vi "Delete Source Files Missing From Install.vi"(8 "Error In":errorcluster, 10 "Source Files":path[](array[path]), 11 "Configuration":T1) -> (0 "Error Out":errorcluster, 2 "Deleted From Souce":path[](array[path]), 3 "Configuration":T1)   [LabVIEW 2011, in "LVH-Build-Tools.lvlib"]
uses:
  LVH-Build-Tools.lvlib
  Type Defs/Configuration.ctl
  Type Defs/Install Configuration.ctl
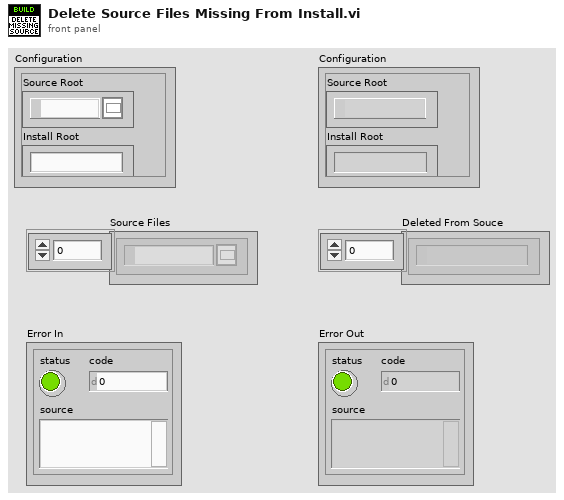
[diagram p1: front panel]
types:
  T1 = typedef "LVH-Build-Tools.lvlib/Configuration.ctl" = cluster{"Source Root":path, "Install Root":string, "Components":string[], "Ignore":string[], "Config Files":path[], "LV Directories":path[], "Install Paths":T2}
  T2 = typedef "LVH-Build-Tools.lvlib/Install Configuration.ctl" = cluster{"LabVIEW Directory":path, "Project Source Config":path}
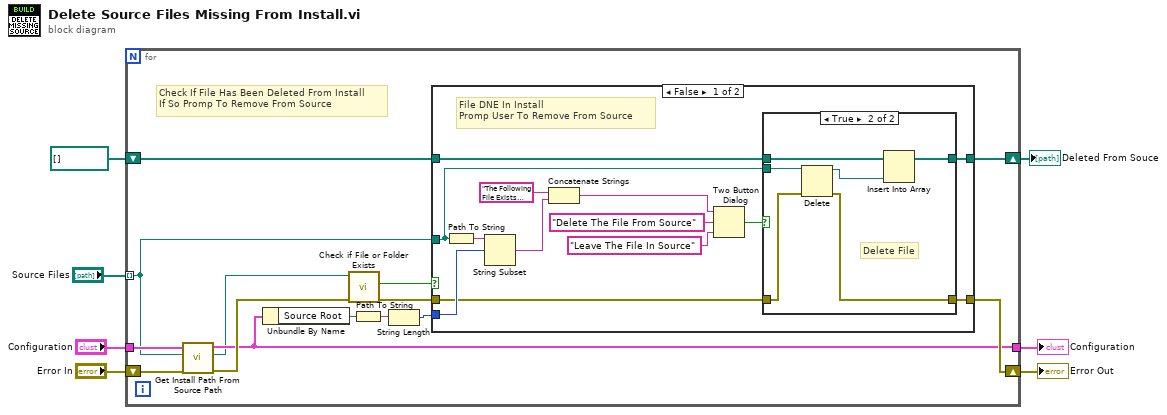
[diagram p0: block diagram]
diagram:
  n1 = for {
    tunnel: "Configuration" -> [w13]
    tunnel: "Source Files" -> [w10] mode=indexing
    shift-right: [w16] -> w7
    shift-left: "Error In" -> [w21]
    tunnel: [w12] -> w1
    shift-right: [w14] -> w6
    shift-left: path[] [] ("Array in") -> [w15]
    # "Check If File Has Been Deleted From Install \nIf So Promp To Remove From Source"
    n2 = call "Get Install Path From Source Path.vi"("Error In"=w21, "Source File Path"=w10, "Configuration"=w13) -> ("Error Out"=w20:errorcluster, "Install File Path"=w11:path, "Configuration"=w12:T1)  [unwired: 5 in, 1 out]
    n3 = Unbundle By Name(w12) -> ("Source Root"=w9:path)
    n4 = call <vilib>:"Check if File or Folder Exists.vi"("error in (no error)"=w20, "path"=w11) -> ("error out"=w18:errorcluster, "file or folder exists?"=w19:bool)  [unwired: 7 in, 1 out]
    n5 = Path To String(path=w9) -> (string=w8:string)
    n6 = String Length(string=w8) -> (length=w17:i32)
    n7 = case shown="False" w19 {
      tunnel: w10 -> [w26 _]
      tunnel: w18 -> [w25 w44]
      tunnel: w17 -> [w32 _]
      tunnel: [w24 w44] -> w16
      tunnel: w15 -> [w23 w43]
      tunnel: [w22 w43] -> w14
      frame False {
        # "File DNE In Install\nPromp User To Remove From Source"
        n8 = Path To String(path=w26) -> (string=w33:string)
        n9 = String Subset(string=w33, offset (0)=w32) -> (substring=w31:string)  [unwired: 1 in]
        n10 = Concatenate Strings("The Following File Exists Under The Source Directory But Not The Install Directory.\n\n", w31) -> (w30:string)
        n11 = Two Button Dialog(message=w30, 1:"Leave The File In Source" ("F button name (\"Cancel\")"), 2:"Delete The File From Source" ("T button name (\"OK\")")) -> (T button?=w27:bool)
        n12 = case shown="True" w27 {
          tunnel: w26 -> [_ w42]
          tunnel: w25 -> [w36 w41]
          tunnel: [w36 w40] -> w24
          tunnel: w23 -> [w35 w39]
          tunnel: [w35 w37] -> w22
          frame False {
            # "Leave File"
          }
          frame True {
            # "Delete File"
            n13 = Delete(path (use dialog)=w42, error in=w41) -> (deleted path=w38:path, error out=w40:errorcluster)  [unwired: 3 in, 1 out]
            n14 = Insert Into Array(array=w39, new element=w38) -> (w37:path[])  [unwired: 1 in]
          }
        }
      }
      frame True {
        # "File Exists In Source And Install.  Move On."
      }
    }
  }
  "Error Out" <- w7
  "Deleted From Souce" <- w6
  "Configuration" <- w1
